vi "Script2d_16x16.vi"() -> ()   [LabVIEW 2011]
uses:
  <vilib>/Utility/miscctls.llb/LVPositionTypeDef.ctl
panel:
  out "Numeric 2":i32
  out "Numeric":i32
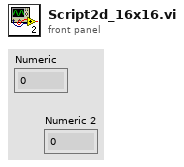
[diagram p1: front panel]
types:
  T1 = enum32{"Invalid", "Standard", "Closed", "Hidden", "Minimized", "Maximized"}
  T2 = typedef "LVPositionTypeDef.ctl" = cluster{"Left":i32, "Top":i32}
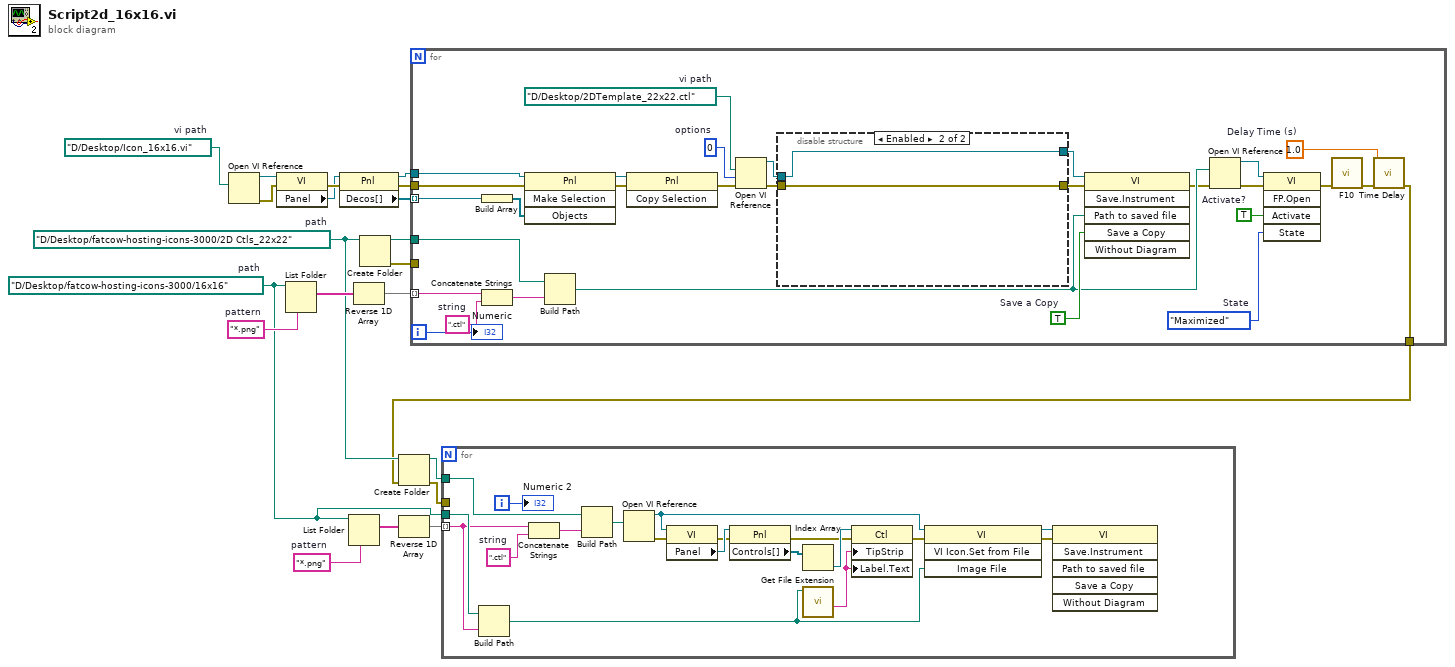
[diagram p0: block diagram]
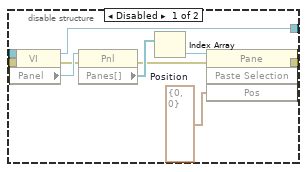
[diagram p2: hidden frame]
diagram:
  w8 = "*.png"  # pattern
  w2 = path "D:/Desktop/fatcow-hosting-icons-3000/2D Ctls_22x22"  # path
  w15 = "*.png"  # pattern
  w3 = path "D:/Desktop/fatcow-hosting-icons-3000/16x16"  # path
  w21 = path "D:/Desktop/Icon_16x16.vi"  # vi path
  n1 = Open VI Reference(vi path=w21) -> (vi reference=w13:refnum<vi>, error out=w12:errorcluster)  [unwired: 5 in]
  n2 = property class="VI"(reference=w13, error in=w12) -> (error out=w19:errorcluster, "Panel"=w16:refnum<vi>)  [unwired: 1 out]
  n3 = List Folder(path=w3, pattern=w15) -> (filenames=w14:string[])  [unwired: 2 in, 3 out]
  n4 = property class="Pnl"(reference=w16, error in=w19) -> (reference out=w18:refnum<vi>, error out=w17:errorcluster, "Decos[]"=w20:refnum<vi>[])
  n5 = List Folder(path=w3, pattern=w8) -> (filenames=w7:string[])  [unwired: 2 in, 3 out]
  n6 = Reverse 1D Array(array=w14) -> (reversed array=w9:string[])
  n7 = Create Folder(path (use dialog)=w2) -> (created path=w11:path, error out=w10:errorcluster)  [unwired: 2 in, 1 out]
  n8 = Reverse 1D Array(array=w7) -> (reversed array=w4:string[])
  n9 = for {
    tunnel: w20 -> [w48] mode=indexing
    tunnel: w18 -> [w45]
    tunnel: w17 -> [w44]
    tunnel: w9 -> [w36] mode=indexing
    tunnel: w11 -> [w33]
    tunnel: w10 -> [_]
    tunnel: [w22] -> w1
    i -> [w23]
    w24 = 1.0  # Delay Time (s)
    w27 = T1."Maximized"  # State
    w29 = TRUE  # Activate?
    w35 = ".ctl"  # string
    w40 = TRUE  # Save a Copy
    w49 = path "D:/Desktop/2DTemplate_22x22.ctl"  # vi path
    w50 = 0  # options
    n10 = Build Array(w48) -> (w37:refnum<vi>[])
    n11 = Concatenate Strings(w36, w35) -> (w34:string)
    n12 = invoke class="Pnl" method="Make Selection"(reference=w45, error in=w44, "Objects"=w37) -> (reference out=w47:refnum<vi>, error out=w43:errorcluster)  [unwired: 1 in, 2 out]
    n13 = Build Path(base path=w33, name or relative path=w34) -> (appended path=w32:path)
    n14 = invoke class="Pnl" method="Copy Selection"(reference=w47, error in=w43) -> (error out=w46:errorcluster)  [unwired: 1 in, 2 out]
    n15 = Open VI Reference(vi path=w49, options=w50, error in (no error)=w46) -> (vi reference=w39:refnum<vi>, error out=w38:errorcluster)  [unwired: 3 in]
    n16 = disable-structure shown="Enabled" {
      disable-tunnel: [w56 w61] -> w42
      disable-tunnel: [w55 w62] -> w41
      disable-tunnel: w39 -> [w53 w61]
      disable-tunnel: w38 -> [w52 w62]
      frame Disabled {
        w57 = T2 {"Left"=0, "Top"=0}  # Position
        n17 = property class="VI"(reference=w53, error in=w52) -> (reference out=w56:refnum<vi>, error out=w58:errorcluster, "Panel"=w59:refnum<vi>)
        n18 = property class="Pnl"(reference=w59, error in=w58) -> (error out=w54:errorcluster, "Panes[]"=w60:refnum<vi>[])  [unwired: 1 out]
        n19 = Index Array(array=w60) -> (element=w51:refnum<vi>)  [unwired: 1 in]
        n20 = invoke class="Pane" method="Paste Selection"(reference=w51, error in=w54, "Pos"=w57) -> (error out=w55:errorcluster)  [unwired: 1 in, 3 out]
      }
      frame Enabled {
      }
    }
    n21 = invoke class="VI" method="Save.Instrument"(reference=w42, error in=w41, "Path to saved file"=w32, "Save a Copy"=w40) -> (error out=w28:errorcluster)  [unwired: 2 in, 5 out]
    n22 = Open VI Reference(vi path=w32, error in (no error)=w28) -> (vi reference=w31:refnum<vi>, error out=w30:errorcluster)  [unwired: 4 in]
    n23 = invoke class="VI" method="FP.Open"(reference=w31, error in=w30, "Activate"=w29, "State"=w27) -> (error out=w26:errorcluster)  [unwired: 1 in, 4 out]
    n24 = call "F10.vi"("error in (no error)"=w26) -> ("error out"=w25:errorcluster)  [unwired: 10 in]
    n25 = call "Time Delay"("error in (no error)"=w25, "Delay Time (s)"=w24) -> ("error out"=w22:errorcluster)  [unwired: 9 in]
    "Numeric" <- w23
  }
  n26 = Create Folder(path (use dialog)=w2, error in=w1) -> (created path=w6:path, error out=w5:errorcluster)  [unwired: 1 in, 1 out]
  n27 = for {
    tunnel: w4 -> [w76] mode=indexing
    tunnel: w6 -> [w79]
    tunnel: w5 -> [_]
    tunnel: w3 -> [w77]
    i -> [w68]
    w81 = ".ctl"  # string
    n28 = Build Path(base path=w77, name or relative path=w76) -> (appended path=w70:path)
    n29 = Concatenate Strings(w76, w81) -> (w80:string)
    n30 = Build Path(base path=w79, name or relative path=w80) -> (appended path=w78:path)
    n31 = Open VI Reference(vi path=w78) -> (vi reference=w74:refnum<vi>, error out=w64:errorcluster)  [unwired: 5 in]
    n32 = property class="VI"(reference=w74, error in=w64) -> (error out=w67:errorcluster, "Panel"=w73:refnum<vi>)  [unwired: 1 out]
    n33 = property class="Pnl"(reference=w73, error in=w67) -> (error out=w66:errorcluster, "Controls[]"=w72:refnum<vi>[])  [unwired: 1 out]
    n34 = Index Array(array=w72) -> (element=w71:refnum<vi>)  [unwired: 1 in]
    n35 = call <vilib>:"Get File Extension.vi"("file"=w70) -> ("filename without extension"=w69:string)  [unwired: 7 in, 3 out]
    n36 = property class="Ctl"(reference=w71, error in=w66, "TipStrip"=w69, "Label.Text"=w69) -> (error out=w65:errorcluster)  [unwired: 1 out]
    n37 = invoke class="VI" method="VI Icon.Set from File"(reference=w74, error in=w65, "Image File"=w70) -> (reference out=w75:refnum<vi>, error out=w63:errorcluster)  [unwired: 1 in, 2 out]
    n38 = invoke class="VI" method="Save.Instrument"(reference=w75, error in=w63) -> ()  [unwired: 4 in, 6 out]
    "Numeric 2" <- w68
  }
